vi "Template Path.vi"(8 "error in (no error)":errorcluster) -> (0 "error out":errorcluster, 3 "path":path)   [LabVIEW 2020]
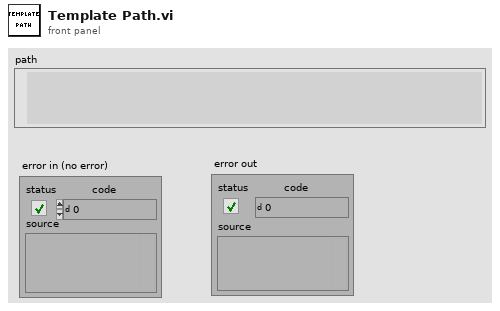
[diagram p1: front panel]
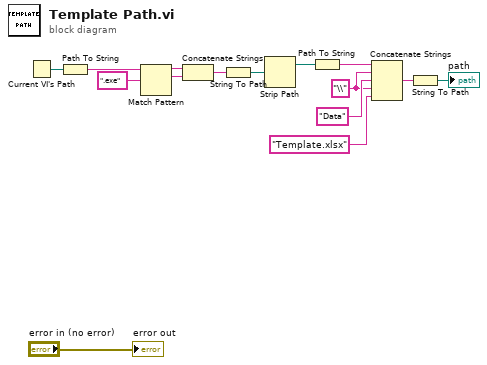
[diagram p0: block diagram]
diagram:
  w6 = "\\" ("string")
  n1 = Current VI's Path() -> (path=w2:path)
  n2 = Path To String(path=w2) -> (string=w15:string)
  n3 = Match Pattern(string=w15, regular expression=".exe") -> (before substring=w13:string, match substring=w12:string)  [unwired: 1 in, 2 out]
  n4 = Concatenate Strings(w13, w12) -> (w11:string)
  n5 = String To Path(string=w11) -> (path=w10:path)
  n6 = Strip Path(path=w10) -> (stripped path=w9:path)  [unwired: 1 out]
  n7 = Path To String(path=w9) -> (string=w8:string)
  n8 = Concatenate Strings(w8, w6, "Data" ("string"), w6, "Template.xlsx" ("string")) -> (w4:string)
  n9 = String To Path(string=w4) -> (path=→"path":path)
  "error out" <- "error in (no error)"
